vi "DAQ-init.vi"() -> (0 "sortie d'erreur":errorcluster, 1 "cluster of DAQ tasks":T1)   [LabVIEW 2015]
uses:
  <vilib>/DAQmx/read.llb/DAQmx Read (Analog 1D DBL 1Chan NSamp).vi
  <vilib>/DAQmx/write.llb/DAQmx Write (Digital Bool 1Line 1Point).vi
  <vilib>/Analysis/baseanly.llb/Mean (DBL).vi
  globalVarSD.vi
  <vilib>/DAQmx/create/channels.llb/DAQmx Create Channel (DO-Digital Output).vi
  <vilib>/DAQmx/create/channels.llb/DAQmx Create Channel (DI-Digital Input).vi
  <vilib>/DAQmx/create/channels.llb/DAQmx Create Channel (AI-Current-Basic).vi
  <vilib>/DAQmx/miscellaneous.llb/DAQmx Fill In Error Info.vi
  <vilib>/Analysis/NI_AALBase.lvlib
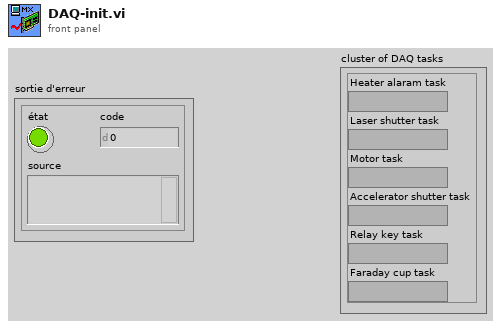
[diagram p1: front panel]
types:
  T1 = cluster{"Heater alaram task":refnum<k21>, "Laser shutter task":refnum<k21>, "Motor task":refnum<k21>, "Accelerator shutter task":refnum<k21>, "Relay key task":refnum<k21>, "Faraday cup task":refnum<k21>}
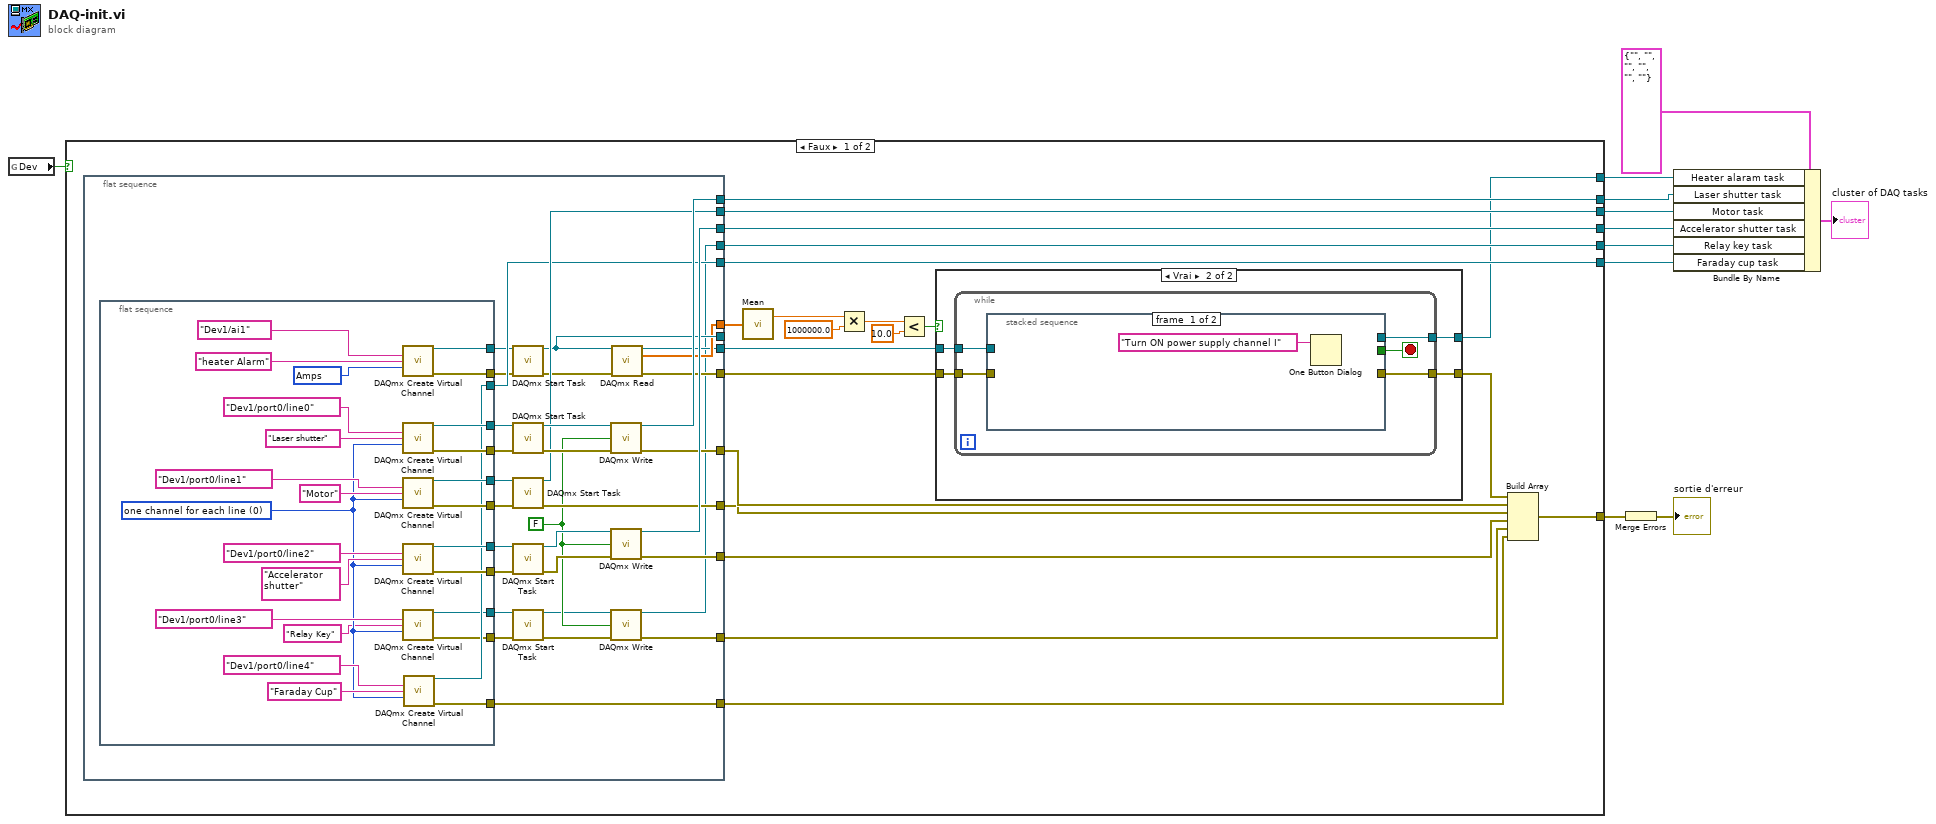
[diagram p0: block diagram]
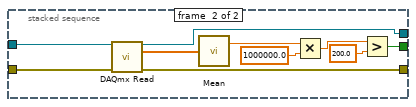
[diagram p3: hidden frame]
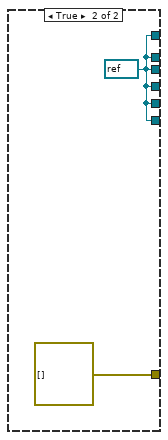
[diagram p4: hidden frame]
diagram:
  n1 = global read "globalVarSD.vi" "Dev"() -> (w11:bool)
  n2 = case shown="Faux" w11 {
    tunnel: [w32 w113] -> w5
    tunnel: [w31 w113] -> w4
    tunnel: [w30 w113] -> w3
    tunnel: [w13 errorcluster[] []] -> w9
    tunnel: [w26 w113] -> w1
    tunnel: [w12 w113] -> w6
    tunnel: [w14 w113] -> w2
    frame False {
      n3 = flat-sequence {
        tunnel: [w60] -> w32
        tunnel: [w57] -> w31
        tunnel: [w52] -> w30
        tunnel: [w51] -> w29
        tunnel: [w50] -> w28
        tunnel: [w49] -> w27
        tunnel: [w48] -> w16
        tunnel: [w47] -> w26
        tunnel: [w44] -> _
        tunnel: [w42] -> w23
        tunnel: [w41] -> w19
        tunnel: [w40] -> w18
        tunnel: [w34] -> w14
        tunnel: [w33] -> w15
        frame #0 {
          w37 = FALSE ("data")
          n4 = flat-sequence {
            tunnel: [w89] -> w64
            tunnel: [w88] -> w63
            tunnel: [w85] -> w59
            tunnel: [w84] -> w58
            tunnel: [w81] -> w56
            tunnel: [w80] -> w55
            tunnel: [w77] -> w48
            tunnel: [w76] -> w47
            tunnel: [w71] -> w46
            tunnel: [w70] -> w45
            tunnel: [w67] -> w38
            tunnel: [w66] -> w39
            frame #0 {
              w68 = 0 items=["one channel for each line", "one channel for all lines"] ("line grouping")
              w73 = 10342 items=["Amps"=10342, "D'une échelle personnalisée"=10065] ("units")
              n5 = call-poly <vilib>:"DAQmx Create Virtual Channel.vi"("physical channels"=tag "Dev1/ai1", "name to assign"="heater Alarm", "units"=w73) -> ("task out"=w71:refnum<k21>, "error out"=w70:errorcluster)  [unwired: 11 in]
              n6 = call-poly <vilib>:"DAQmx Create Virtual Channel.vi"("lines"=tag "Dev1/port0/line0" ("Lines"), "name to assign"="Laser shutter", "line grouping"=w68) -> ("task out"=w88:refnum<k21>, "error out"=w89:errorcluster)  [unwired: 11 in]
              n7 = call-poly <vilib>:"DAQmx Create Virtual Channel.vi"("lines"=tag "Dev1/port0/line1" ("Lines"), "name to assign"="Motor", "line grouping"=w68) -> ("task out"=w85:refnum<k21>, "error out"=w84:errorcluster)  [unwired: 11 in]
              n8 = call-poly <vilib>:"DAQmx Create Virtual Channel.vi"("lines"=tag "Dev1/port0/line2" ("Lines"), "name to assign"="Accelerator shutter", "line grouping"=w68) -> ("task out"=w80:refnum<k21>, "error out"=w81:errorcluster)  [unwired: 11 in]
              n9 = call-poly <vilib>:"DAQmx Create Virtual Channel.vi"("lines"=tag "Dev1/port0/line3" ("Lines"), "name to assign"="Relay Key", "line grouping"=w68) -> ("task out"=w66:refnum<k21>, "error out"=w67:errorcluster)  [unwired: 11 in]
              n10 = call-poly <vilib>:"DAQmx Create Virtual Channel.vi"("lines"=tag "Dev1/port0/line4" ("Lines"), "name to assign"="Faraday Cup", "line grouping"=w68) -> ("task out"=w76:refnum<k21>, "error out"=w77:errorcluster)  [unwired: 11 in]
            }
          }
          n11 = call <vilib>:"DAQmx Start Task.vi"("task/channels in"=w46, "error in"=w45) -> ("task out"=w44:refnum<k21>, "error out"=w43:errorcluster)  [unwired: 12 in]
          n12 = call <vilib>:"DAQmx Start Task.vi"("task/channels in"=w63, "error in"=w64) -> ("task out"=w62:refnum<k21>, "error out"=w61:errorcluster)  [unwired: 12 in]
          n13 = call <vilib>:"DAQmx Start Task.vi"("task/channels in"=w59, "error in"=w58) -> ("task out"=w57:refnum<k21>, "error out"=w50:errorcluster)  [unwired: 12 in]
          n14 = call <vilib>:"DAQmx Start Task.vi"("task/channels in"=w55, "error in"=w56) -> ("task out"=w54:refnum<k21>, "error out"=w53:errorcluster)  [unwired: 12 in]
          n15 = call <vilib>:"DAQmx Start Task.vi"("task/channels in"=w39, "error in"=w38) -> ("task out"=w36:refnum<k21>, "error out"=w35:errorcluster)  [unwired: 12 in]
          n16 = call-poly <vilib>:"DAQmx Write.vi"("task/channels in"=w62, "data"=w37, "error in"=w61) -> ("task out"=w60:refnum<k21>, "error out"=w51:errorcluster)  [unwired: 10 in, 1 out]
          n17 = call-poly <vilib>:"DAQmx Write.vi"("task/channels in"=w54, "data"=w37, "error in"=w53) -> ("task out"=w52:refnum<k21>, "error out"=w49:errorcluster)  [unwired: 10 in, 1 out]
          n18 = call-poly <vilib>:"DAQmx Write.vi"("task/channels in"=w36, "data"=w37, "error in"=w35) -> ("task out"=w34:refnum<k21>, "error out"=w33:errorcluster)  [unwired: 10 in, 1 out]
          n19 = call-poly <vilib>:"DAQmx Read.vi"("task/channels in"=w44, "error in"=w43) -> ("task out"=w41:refnum<k21>, "data"=w42:dbl[], "error out"=w40:errorcluster)  [unwired: 11 in]
        }
      }
      n20 = call-poly <vilib>:"Mean.vi"("X"=w23) -> ("mean"=w25:dbl)  [unwired: 1 out]
      n21 = Multiply(x=w25, y=1000000.0) -> (x*y=w22:dbl)
      n22 = Less?(x=w22, y=10.0) -> (x < y?=w20:bool)
      n23 = case shown="Vrai" w20 {
        tunnel: w19 -> [w91 w96]
        tunnel: w18 -> [w92 w95]
        tunnel: [w92 w94] -> w17
        tunnel: [w91 w93] -> w12
        frame False {
        }
        frame True {
          n24 = while {
            tunnel: w96 -> [w101]
            tunnel: w95 -> [w99]
            tunnel: [w98] -> w94
            tunnel: [w97] -> w93
            stop <- w100 stop-if-true
            n25 = stacked-sequence {
              tunnel: w101 -> [_ w112]
              tunnel: [_ w108] -> w100
              tunnel: w99 -> [_ w105]
              tunnel: [_ w104] -> w98
              tunnel: [_ w103] -> w97
              frame #0 {
                n26 = One Button Dialog(message="Turn ON power supply channel I") -> ()  [unwired: 1 in, 1 out]
              }
              frame #1 {
                n27 = call-poly <vilib>:"DAQmx Read.vi"("task/channels in"=w112, "error in"=w105) -> ("task out"=w103:refnum<k21>, "data"=w107:dbl[], "error out"=w104:errorcluster)  [unwired: 11 in]
                n28 = call-poly <vilib>:"Mean.vi"("X"=w107) -> ("mean"=w106:dbl)  [unwired: 1 out]
                n29 = Multiply(x=w106, y=1000000.0) -> (x*y=w110:dbl)
                n30 = Greater?(x=w110, y=200.0) -> (0:w108:bool)
              }
            }
          }
        }
      }
      n31 = Build Array(w17, w29, w28, w27, w15, w16) -> (w13:errorcluster[])
    }
    frame True {
      w113 = refnum<k21> refnum ("task out")
    }
  }
  n32 = Merge Errors(w9) -> (→"sortie d'erreur":errorcluster)
  n33 = Bundle By Name(cluster=T1 {"Heater alaram task"="", "Laser shutter task"="", "Motor task"="", "Accelerator shutter task"="", "Relay key task"="", "Faraday cup task"=""} ("cluster d'entrée"), "Heater alaram task"=w6, "Laser shutter task"=w5, "Motor task"=w4, "Accelerator shutter task"=w3, "Relay key task"=w2, "Faraday cup task"=w1) -> (→"cluster of DAQ tasks":T1)
